vi "movSPEX.vi"(10 "longitud de onda":dbl) -> (2 "Lamda":dbl)   [LabVIEW 2016]
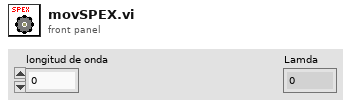
[diagram p1: front panel]
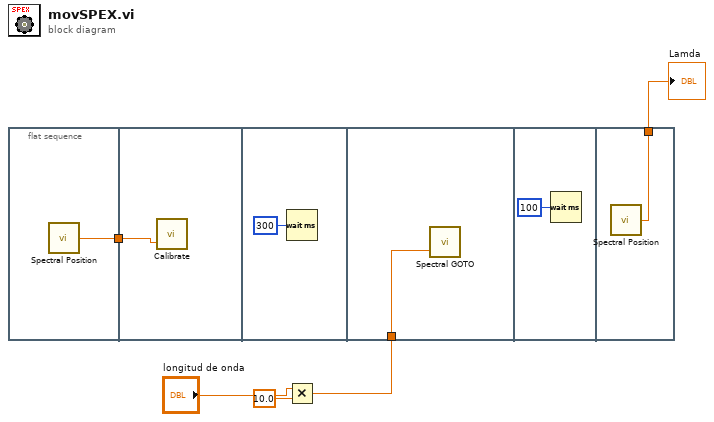
[diagram p0: block diagram]
diagram:
  n1 = flat-sequence {
    tunnel: [w6] -> w5
    tunnel: w5 -> [w7]
    tunnel: w2 -> [w9]
    tunnel: [w11] -> w4
    frame #0 {
      n2 = call "Spectral Position.VI"() -> ("Present Position"=w6:dbl)  [unwired: 1 in, 2 out]
    }
    frame #1 {
      n3 = call "Calibrate.VI"("Counter Position"=w7) -> ()  [unwired: 1 in, 3 out]
    }
    frame #2 {
      n4 = Wait (ms)(milliseconds to wait=u32 300) -> ()  [unwired: 1 out]
    }
    frame #3 {
      n5 = call "Spectral GOTO.VI"("Target Position"=w9) -> ()  [unwired: 1 in, 3 out]
    }
    frame #4 {
      n6 = Wait (ms)(milliseconds to wait=u32 100) -> ()  [unwired: 1 out]
    }
    frame #5 {
      n7 = call "Spectral Position.VI"() -> ("Present Position"=w11:dbl)  [unwired: 1 in, 2 out]
    }
  }
  n8 = Multiply(x="longitud de onda", y=10.0) -> (x*y=w2:dbl)
  "Lamda" <- w4
